vi "appendText.vi"(8 "error in (no error)":errorcluster, 9 "Style":refnum<class "Style.lvclass">, 10 "Text":string, 11 "MS-Word in":refnum<class "MS-Word.lvclass">) -> (0 "error out":errorcluster, 3 "MS-Word out":refnum<class "MS-Word.lvclass">)   [LabVIEW 2017, in "LabVIEW NPOI.lvlib" / "MS-Word.lvclass"]
uses:
  MS-Word.lvclass
  Styles/Style/Style.lvclass
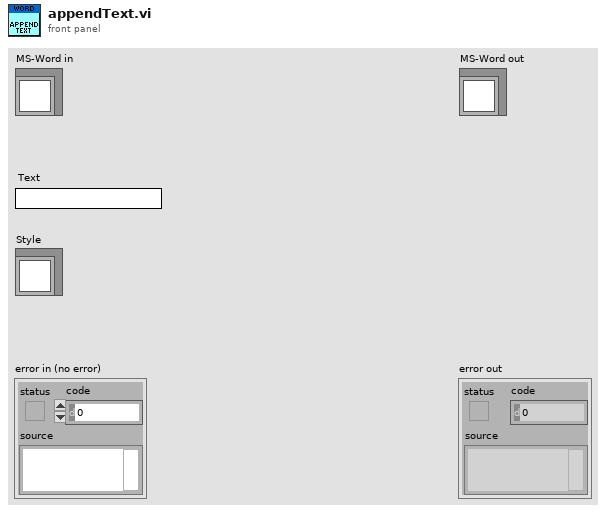
[diagram p1: front panel]
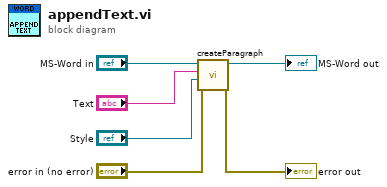
[diagram p0: block diagram]
diagram:
  n1 = call-dynamic "createParagraph.vi"("error in (no error)"="error in (no error)", "Style"="Style", "Text"="Text", "MS-Word in"="MS-Word in") -> ("error out"=→"error out":errorcluster, "MS-Word out"=→"MS-Word out":refnum<class "MS-Word.lvclass">)  [unwired: 6 in]
